vi "Send StageMoveDone.vi"(7 "Message Priority (Normal)":T2=enum."Normal", 8 "error in (no error)":errorcluster, 10 "Positions":T1={"CH1 Pos"=0, "CH2 Pos"=0, "CH3 Pos"=0, "CH4 Pos"=0, "Home?"=TRUE}, 11 "Message Enqueuer":refnum<class "Message Enqueuer.lvclass">) -> (0 "error out":errorcluster, 3 "Message Enqueuer out":refnum<class "Message Enqueuer.lvclass">)   [LabVIEW 2023, in "StageMoveDone Msg.lvclass"]
doc: "This VI sends the message to an actor."
uses:
  StageMoveDone Msg.lvclass
  StageMoveDone Msg.lvclass/StageMoveDone Msg.ctl
  <vilib>/ActorFramework/Message Enqueuer/Message Enqueuer.lvclass
  C:/Program Files/National Instruments/LabVIEW 2023/vi.lib/ActorFramework/Message/Message.lvclass
  C:/Users/quantum/Documents/LVDAQ/UIs/TranslationStage_UI/TranslationStage_UI Messages/StageMoveDone Msg/StageMoveDone Msg.lvclass
  <vilib>/ActorFramework/Message Enqueuer/Message Priority.ctl
  TranslationStage_UI/StageMoveDone_For_UI.ctl
  typedefs/typedefs.lvlib
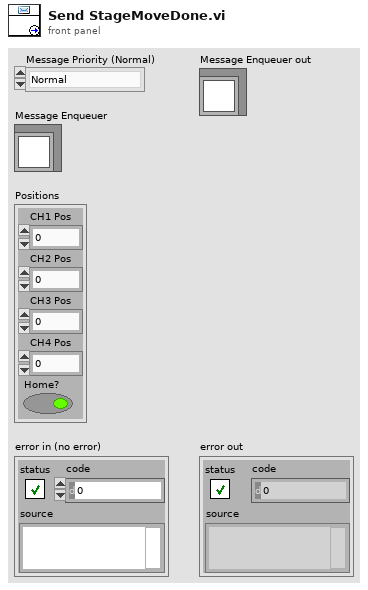
[diagram p1: front panel]
types:
  T1 = typedef "typedefs.lvlib/StageMoveDone_For_UI.ctl" = cluster{"CH1 Pos":i32, "CH2 Pos":i32, "CH3 Pos":i32, "CH4 Pos":i32, "Home?":bool}
  T2 = typedef "Actor Framework.lvlib/Message Enqueuer.lvclass/Message Priority.ctl" = enum16{"Low", "Normal", "High"}
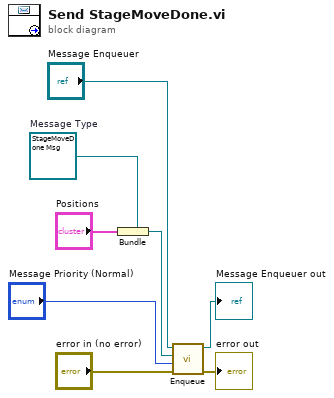
[diagram p0: block diagram]
diagram:
  w5 = refnum<class "StageMoveDone Msg.lvclass"> refnum  # Message Type
  n1 = Bundle(cluster=w5, "Positions") -> (w4:refnum<class "StageMoveDone Msg.lvclass">)
  n2 = call <vilib>:"Enqueue.vi"("error in (no error)"="error in (no error)", "Message Priority (Normal)"="Message Priority (Normal)", "Message"=w4, "Message Enqueuer in"="Message Enqueuer") -> ("error out"=→"error out":errorcluster, "Message Enqueuer in"=→"Message Enqueuer out":refnum<class "Message Enqueuer.lvclass">)  [unwired: 6 in]
